vi "ProjectSilentDisconnect.vi"(9 "Undeploy System Definition (F)":bool, 10 "Password (\"\")":string, 11 "Gateway IP Address (\"\": localhost)":string) -> (0 "error out":errorcluster)   [LabVIEW 2020, in "ni-veristand-steps-runtime-lib.lvlib"]
uses:
  ni-veristand-steps-runtime-lib.lvlib
  <vilib>/NI VeriStand/Execution/Workspace/NI_VS Workspace ExecutionAPI.lvlib
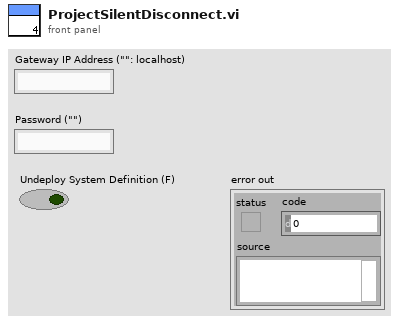
[diagram p1: front panel]
types:
  T1 = typedef "NI_VS Workspace ExecutionAPI.lvlib/WorkspaceAPI.ctl" = refnum<k24>
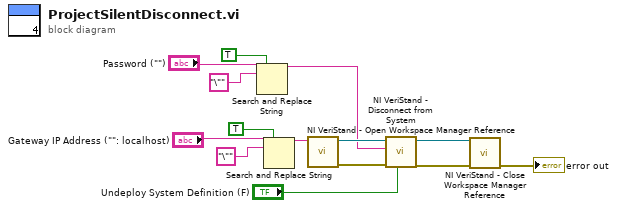
[diagram p0: block diagram]
diagram:
  n1 = Search and Replace String(replace all?=TRUE ("replace all? (F)"), input string="Password (\"\")", search string="\"") -> (result string=w1:string)  [unwired: 5 in, 3 out]
  n2 = Search and Replace String(replace all?=TRUE ("replace all? (F)"), input string="Gateway IP Address (\"\": localhost)", search string="\"") -> (result string=w6:string)  [unwired: 5 in, 3 out]
  n3 = call <vilib>:"NI VeriStand - Open Workspace Manager Reference.vi"("Gateway IP Address (\"\": localhost)"=w6) -> ("error out"=w14:errorcluster, "WorkspaceManager"=w13:T1)  [unwired: 9 in]
  n4 = call <vilib>:"NI VeriStand - Disconnect from System.vi"("Undeploy System Definition (F)"="Undeploy System Definition (F)", "error in (no error)"=w14, "Password (\"\")"=w1, "WorkspaceManager in"=w13) -> ("error out"=w11:errorcluster, "WorkspaceManager out"=w10:T1)  [unwired: 6 in]
  n5 = call <vilib>:"NI VeriStand - Close Workspace Manager Reference.vi"("error in (no error)"=w11, "WorkspaceManager"=w10) -> ("error out"=→"error out":errorcluster)  [unwired: 9 in]
